vi "Stepper_Sub.vi"(9 "Anzahl Schritte":dbl=1000.0, 10 "Schritte/Umdrehung":dbl=100.0, 11 "Geschwindigkeit":dbl) -> (2 "error out":errorcluster={"status"=FALSE, "code"=1073676294, "source"="VISA Read in LabVIEW Interface for Arduino.lvlib:Send Receive.vi->Stepper_Sub.vi"}, 3 "Arduino Resource 2":T1={"VISA resource"="COM10", "Board Type"=enum."Mega 2560", "Connection Type"=enum."USB / Serial", "Bytes Per Packet (15)"=15})   [LabVIEW 2013]
uses:
  <vilib>/LabVIEW Interface for Arduino/Type Defs/Arduino Resource.ctl
  <vilib>/LabVIEW Interface for Arduino/Type Defs/Board Type.ctl
  <vilib>/LabVIEW Interface for Arduino/Type Defs/Pin Mode.ctl
  <vilib>/LabVIEW Interface for Arduino/LabVIEW Interface for Arduino.lvlib
panel:
  in  "Richtung":bool=TRUE
  out "Numeric":i32=99
  out "appended array":u8[](array[numeric])=[253, 3, 8]
  out "subarray":bool[](array[boolean])=[FALSE, FALSE, FALSE, TRUE]
  in  "disabled index (col) 2":i32=1
  in  "Array 2":bool[][](array[boolean])=[[TRUE, FALSE, FALSE, TRUE, TRUE, FALSE, FALSE, FALSE], [FALSE, TRUE, TRUE, FALSE, FALSE, TRUE, TRUE, FALSE], [TRUE, TRUE, FALSE, FALSE, TRUE, TRUE, FALSE, FALSE], [FALSE, FALSE, TRUE, TRUE, FALSE, FALSE, TRUE, TRUE], [FALSE, FALSE, FALSE, FALSE, FALSE, FALSE, FALSE, FALSE], [FALSE, FALSE, FALSE, FALSE, FALSE, FALSE, FALSE, FALSE], [FALSE, FALSE, FALSE, FALSE, FALSE, FALSE, FALSE, FALSE], [FALSE, FALSE, FALSE, FALSE, FALSE, FALSE, FALSE, FALSE]]
  out "Numeric 2":i32=7
  in  "Digital I/O Pin 5":u8=6
  in  "Digital I/O Pin 4":u8=5
  in  "Digital I/O Pin 3":u8=4
  in  "Digital I/O Pin 2":u8=3
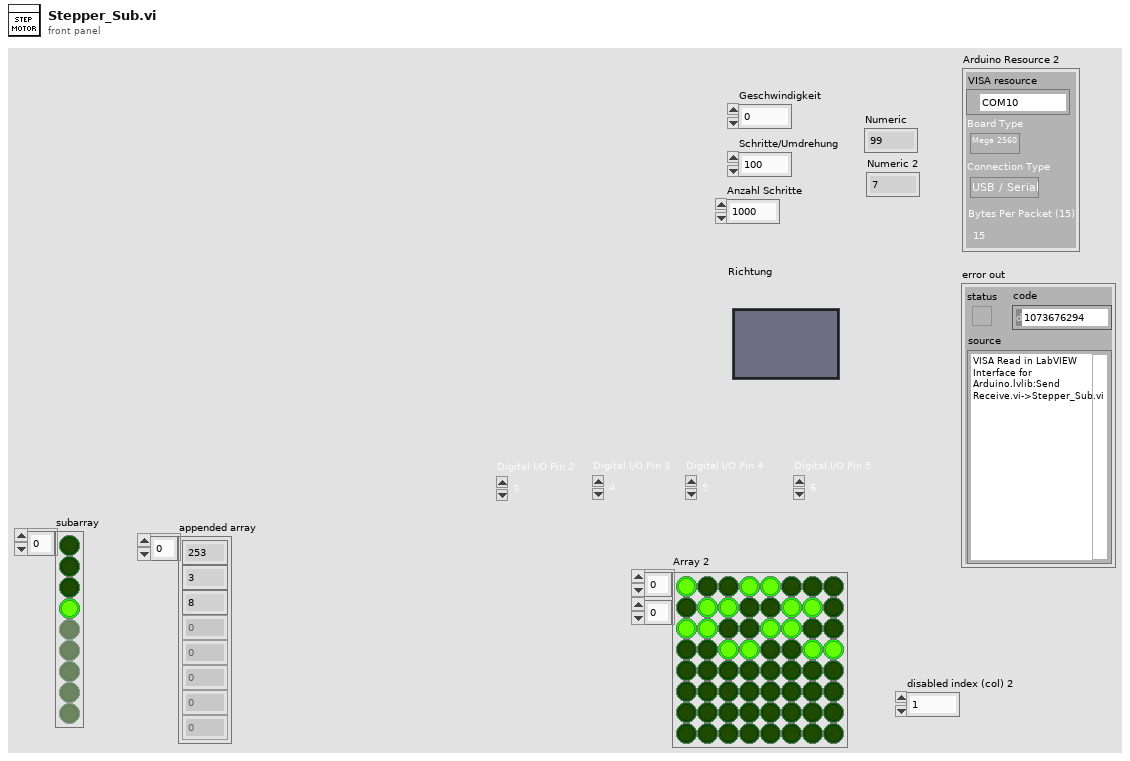
[diagram p1: front panel]
types:
  T1 = typedef "LabVIEW Interface for Arduino.lvlib/Arduino Resource.ctl" = cluster{"VISA resource":refnum<visa-resource-name>, "Board Type":T2, "Connection Type":enum8{"USB / Serial"}, "Bytes Per Packet (15)":u8}
  T2 = typedef "LabVIEW Interface for Arduino.lvlib/Board Type.ctl" = enum16{"Uno", "Dimuelanove w/Atmega 328", "Mega 2560"}
  T3 = typedef "LabVIEW Interface for Arduino.lvlib/Pin Mode.ctl" = enum8{"Input", "Output"}
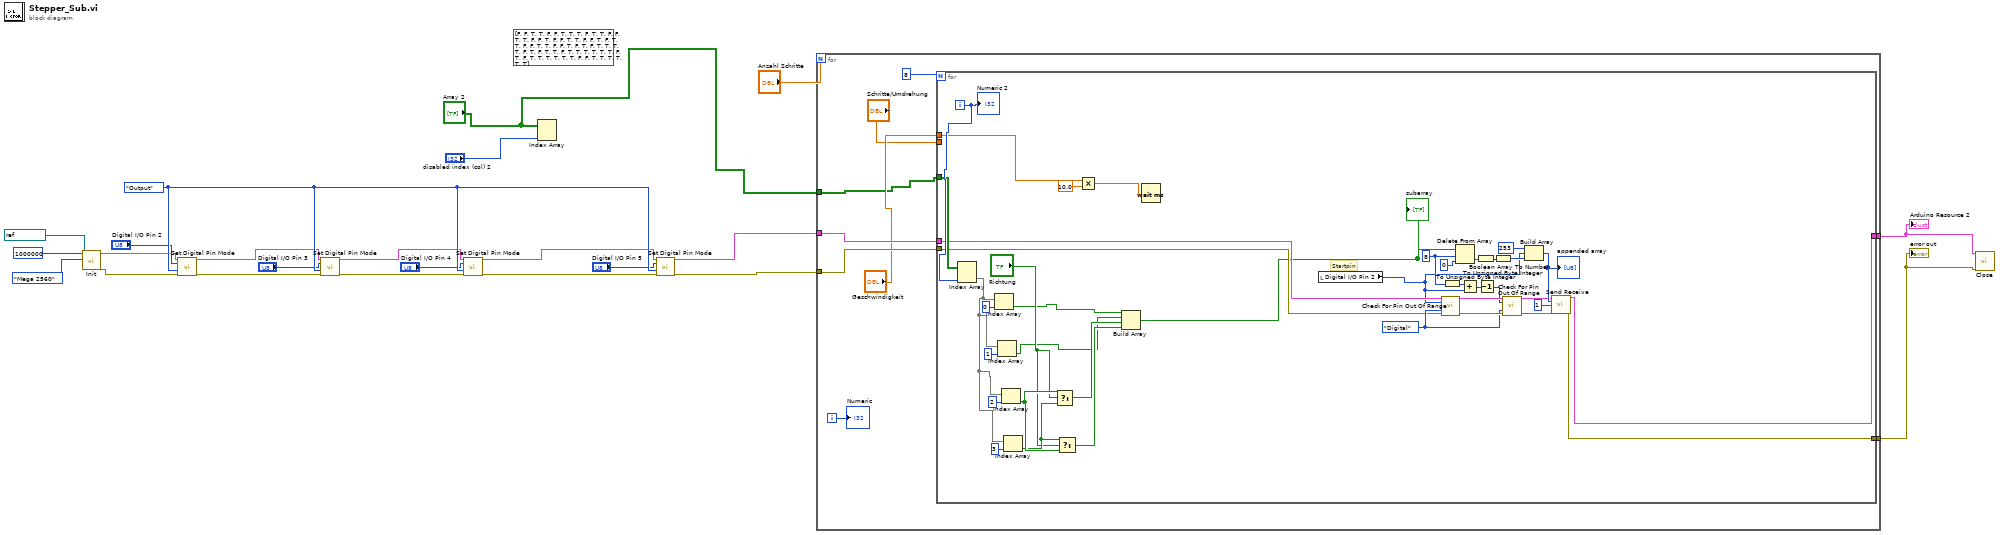
[diagram p0: block diagram]
diagram:
  w23 = Pin_Mode."Output" ("Pin Mode (Input)")
  (unwired) bool[][] [[FALSE, FALSE, TRUE, TRUE, FALSE, FALSE, TRUE, TRUE, TRUE], [FALSE, TRUE, TRUE, FALSE, FALSE, TRUE, TRUE, FALSE, FALSE], [TRUE, FALSE, FALSE, TRUE, TRUE, FALSE, FALSE, TRUE, FALSE], [TRUE, TRUE, FALSE, FALSE, TRUE, TRUE, FALSE, FALSE, TRUE], [FALSE, TRUE, FALSE, TRUE, TRUE, TRUE, TRUE, FALSE, TRUE], [FALSE, TRUE, TRUE, FALSE, TRUE, TRUE, TRUE, TRUE, TRUE], [TRUE, FALSE, TRUE, FALSE, TRUE, TRUE, TRUE, TRUE, TRUE], [TRUE, FALSE, FALSE, TRUE, TRUE, TRUE, TRUE, TRUE, TRUE]]
  n1 = call <vilib>:"Init.vi"("VISA resource"=refnum<visa-resource-name> "COM10", "Baud Rate (115200)"=u32 1000000, "Board Type (Uno)"=Board_Type."Mega 2560") -> ("Arduino Resource"=w3:T1, "error out"=w5:errorcluster)  [unwired: 15 in]
  n2 = call <vilib>:"Set Digital Pin Mode.vi"("Arduino Resource"=w3, "Digital I/O Pin"="Digital I/O Pin 2", "Pin Mode (Input)"=w23, "error in"=w5) -> ("Arduino Resource"=w22:T1, "error out"=w19:errorcluster)  [unwired: 10 in]
  n3 = call <vilib>:"Set Digital Pin Mode.vi"("Arduino Resource"=w22, "Digital I/O Pin"="Digital I/O Pin 3", "Pin Mode (Input)"=w23, "error in"=w19) -> ("Arduino Resource"=w21:T1, "error out"=w18:errorcluster)  [unwired: 10 in]
  n4 = call <vilib>:"Set Digital Pin Mode.vi"("Arduino Resource"=w21, "Digital I/O Pin"="Digital I/O Pin 4", "Pin Mode (Input)"=w23, "error in"=w18) -> ("Arduino Resource"=w20:T1, "error out"=w17:errorcluster)  [unwired: 10 in]
  n5 = Index Array(array="Array 2", index (col)="disabled index (col) 2") -> ()  [unwired: 1 in, 1 out]
  n6 = call <vilib>:"Set Digital Pin Mode.vi"("Arduino Resource"=w20, "Digital I/O Pin"="Digital I/O Pin 5", "Pin Mode (Input)"=w23, "error in"=w17) -> ("Arduino Resource"=w12:T1, "error out"=w11:errorcluster)  [unwired: 10 in]
  n7 = for {
    N: "Anzahl Schritte" -> [_]
    tunnel: w12 -> [w31]
    tunnel: w11 -> [w30]
    tunnel: "Array 2" -> [w24]
    tunnel: [w27] -> w1
    tunnel: [w26] -> w2
    i -> [w25]
    n8 = for {
      N: 8 -> [_]
      tunnel: w24 -> [w70]
      tunnel: "Schritte/Umdrehung" -> [_]
      tunnel: "Geschwindigkeit" -> [w62]
      tunnel: w31 -> [w44]
      tunnel: w30 -> [w43]
      tunnel: [w42] -> w26
      tunnel: [w41] -> w27
      i -> [w71]
      w50 = enum16{"Analog", "Digital"}."Digital" ("Pin Type")
      w48 = 8 ("length")
      # "Startpin"
      n9 = Index Array(array=w70, index (col)=w71) -> (element=w39:bool[])  [unwired: 1 in]
      n10 = Index Array(array=w39, index=0) -> (element=w33:bool)
      n11 = Index Array(array=w39, index=1) -> (element=w34:bool)
      n12 = Index Array(array=w39, index=2) -> (element=w38:bool)
      n13 = Index Array(array=w39, index=3) -> (element=w37:bool)
      n14 = Select(t=w38, s="Richtung", f=w37) -> (s? t:f=w65:bool)
      n15 = Select(t=w37, s="Richtung", f=w38) -> (s? t:f=w64:bool)
      n16 = Multiply(x=w62, y=10.0) -> (x*y=w63:dbl)
      n17 = Build Array(w33, w34, w65, w64) -> (w35:bool[])
      "subarray" <- w35
      n18 = Wait (ms)(milliseconds to wait=w63) -> ()  [unwired: 1 out]
      n19 = local read "Digital I/O Pin 2"() -> (w40:u8)
      n20 = call <vilib>:"Check For Pin Out Of Range.vi"("Arduino Resource"=w44, "User Pin Number"=w40, "Pin Type"=w50, "error in"=w43) -> ("Arduino Resource"=w54:T1, "error out"=w53:errorcluster)  [unwired: 10 in]
      n21 = To Unsigned Byte Integer(number=w48) -> (unsigned 8bit integer=w47:u8)
      n22 = Delete From Array(array=w35, length=w48, index=0) -> (deleted portion=w56:bool[])  [unwired: 1 out]
      n23 = Add(x=w47, y=w40) -> (x+y=w49:u8)
      n24 = Boolean Array To Number(Boolean array=w56) -> (number=w57:u32)
      n25 = Decrement(x=w49) -> (x-1=w46:u8)
      n26 = To Unsigned Byte Integer(number=w57) -> (unsigned 8bit integer=w45:u8)
      n27 = call <vilib>:"Check For Pin Out Of Range.vi"("Arduino Resource"=w54, "User Pin Number"=w46, "Pin Type"=w50, "error in"=w53) -> ("Arduino Resource"=w51:T1, "error out"=w52:errorcluster)  [unwired: 10 in]
      n28 = Build Array(u8 253, w40, w45) -> (w60:u8[])
      "appended array" <- w60
      n29 = call <vilib>:"Send Receive.vi"("Arduino Resource"=w51, "Data"=w60, "Bytes To Read (0)"=u32 1, "error in"=w52) -> ("Arduino Resource"=w42:T1, "error out"=w41:errorcluster)  [unwired: 9 in, 1 out]
      "Numeric 2" <- w71
    }
    "Numeric" <- w25
  }
  "error out" <- w1
  "Arduino Resource 2" <- w2
  n30 = call <vilib>:"Close.vi"("Arduino Resource"=w2, "error in"=w1) -> ()  [unwired: 13 in, 1 out]
